vi "Gear_Components.vi"(9 "Target Seperation":dbl, 10 "Far Target Distance":dbl, 11 "Close Target Distance":dbl) -> (2 "X Component":dbl, 3 "Y Component":dbl)   [LabVIEW 2016]
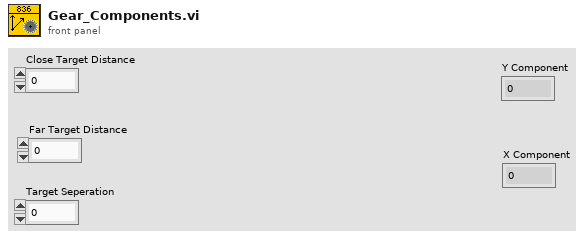
[diagram p1: front panel]
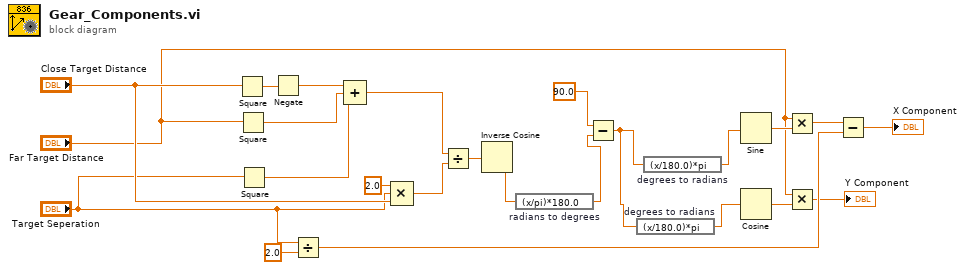
[diagram p0: block diagram]
diagram:
  n1 = Square(x="Close Target Distance") -> (x^2=w23:dbl)
  n2 = Square(x="Far Target Distance") -> (x^2=w22:dbl)
  n3 = Square(x="Target Seperation") -> (x^2=w21:dbl)
  n4 = Negate(x=w23) -> (-x=w6:dbl)
  n5 = Divide(x="Target Seperation", y=2.0) -> (x/y=w11:dbl)
  n6 = Compound Arithmetic op=ADD(w6, w22, w21) -> (w20:dbl)
  n7 = Compound Arithmetic op=MULTIPLY(2.0 ("value"), "Target Seperation", "Close Target Distance") -> (w17:dbl)
  n8 = Divide(x=w20, y=w17) -> (x/y=w24:dbl)
  n9 = Inverse Cosine(1:w24) -> (0:w5:dbl)
  n10 = expression code="(x/pi)*180.0" "radians to degrees"(w5) -> (w4:dbl)
  n11 = Subtract(x=90.0, y=w4) -> (x-y=w2:dbl)
  n12 = expression code="(x/180.0)*pi" "degrees to radians"(w2) -> (w3:dbl)
  n13 = expression code="(x/180.0)*pi" "degrees to radians"(w2) -> (w1:dbl)
  n14 = Sine(x=w1) -> (sin(x)=w15:dbl)
  n15 = Cosine(x=w3) -> (cos(x)=w9:dbl)
  n16 = Multiply(x="Far Target Distance", y=w15) -> (x*y=w14:dbl)
  n17 = Multiply(x="Far Target Distance", y=w9) -> (x*y=→"Y Component":dbl)
  n18 = Subtract(x=w14, y=w11) -> (x-y=→"X Component":dbl)
